vi "Main OOB Comm.vi"(8 "error in":errorcluster, 10 "gRPC to Main":T2, 11 "Node in":refnum<class "AMS Cycler Template.lvclass">) -> (0 "error out":errorcluster, 1 "Update":bool, 2 "Main to gRPC":T1, 3 "Node out":refnum<class "AMS Cycler Template.lvclass">)   [LabVIEW 2023, in "AMS Cycler Template.lvlib" / "AMS Cycler Template.lvclass"]
uses:
  AMS Cycler Template.lvclass
  Type Defs/gRPC to Main.ctl
  Type Defs/Main to gRPC.ctl
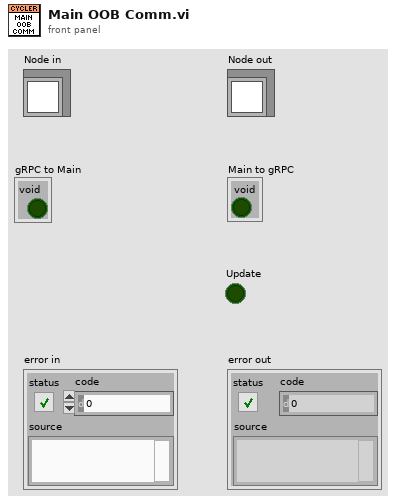
[diagram p1: front panel]
types:
  T1 = typedef "AMS Cycler Template.lvlib/AMS Cycler Template.lvclass/Main to gRPC.ctl" = cluster{"void":bool}
  T2 = typedef "AMS Cycler Template.lvlib/AMS Cycler Template.lvclass/gRPC to Main.ctl" = cluster{"void":bool}
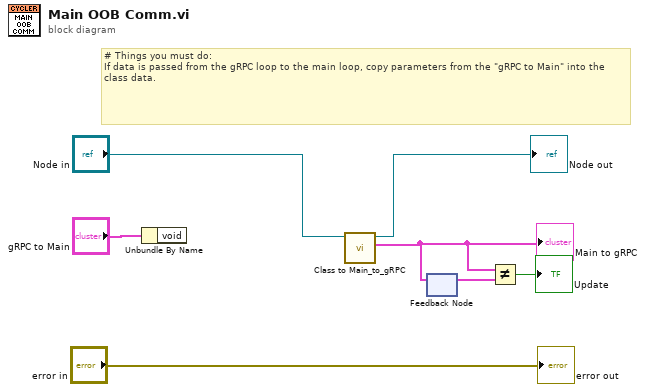
[diagram p0: block diagram]
diagram:
  # "# Things you must do:\nIf data is passed from the gRPC loop to the main loop, copy parameters from the \"gRPC to Main\" into the class data."
  n1 = Unbundle By Name("gRPC to Main") -> ()  [unwired: 1 out]
  n2 = call "Class to Main_to_gRPC.vi"("Timed Node in"="Node in") -> ("Main to gRPC"=w2:T1, "Timed Node out"=→"Node out":refnum<class "AMS Cycler Template.lvclass">)  [unwired: 9 in]
  "Main to gRPC" <- w2
  n3 = feedback #1() -> (w7:T1)  [unwired: 1 in]
  n4 = feedback-in #1(w2) -> ()
  n5 = Not Equal?(x=w2, y=w7) -> (x != y?=→"Update":bool)
  "error out" <- "error in"
